vi "Get SMO Database Paths.vi"(5 "getAll Cluster":variant, 7 "Default Paths":string, 8 "error in (no error)":errorcluster, 11 "instrument.PPMS in":refnum<class "instrument.PPMS1.lvclass">) -> (0 "error out":errorcluster, 2 "Paths":string, 3 "instrument.PPMS out":refnum<class "instrument.PPMS1.lvclass">)   [LabVIEW 2019, in "instrument.PPMS1.lvclass"]
uses:
  instrument.PPMS1.lvclass
  instrument.PPMS/instrument.PPMS.lvclass
  instrument.PPMS/Typedefs/PPMS.getAll--cluster.ctl
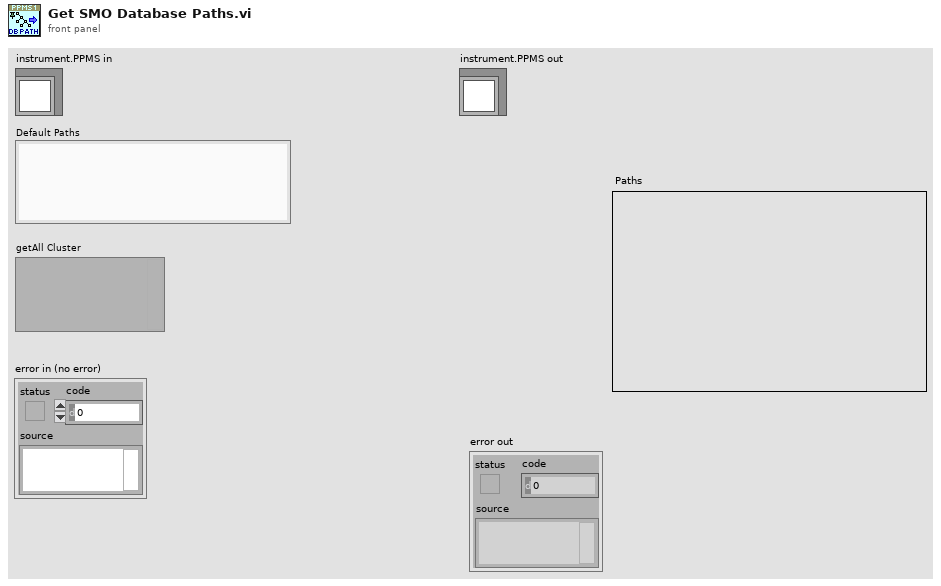
[diagram p1: front panel]
types:
  T1 = typedef "instrument.PPMS.lvclass/PPMS.getAll--cluster.ctl" = cluster{"Chamber Status":string, "Helium Level":dbl, "Temperature":dbl, "Temperature Status":string, "Magnetic Field":dbl, "Magnet Status":string, "Position":dbl}
  T2 = cluster{"Chamber Status":string, "Helium Level":dbl, "Temperature":dbl, "Temperature Status":string, "Magnetic Field":dbl, "Magnet Status":string}
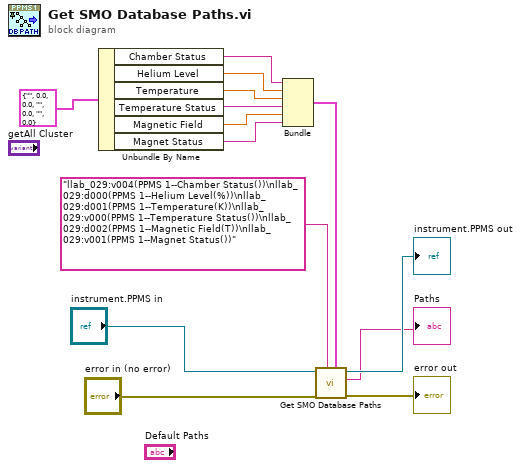
[diagram p0: block diagram]
diagram:
  n1 = Unbundle By Name(T1 {"Chamber Status"="", "Helium Level"=0.0, "Temperature"=0.0, "Temperature Status"="", "Magnetic Field"=0.0, "Magnet Status"="", "Position"=0.0} ("getAll")) -> ("Chamber Status"=w2:string, "Helium Level"=w5:dbl, "Temperature"=w6:dbl, "Temperature Status"=w7:string, "Magnetic Field"=w4:dbl, "Magnet Status"=w3:string)
  n2 = Bundle("Chamber Status"=w2, "Helium Level"=w5, "Temperature"=w6, "Temperature Status"=w7, "Magnetic Field"=w4, "Magnet Status"=w3) -> (w1:T2)  [unwired: 1 in]
  n3 = call-parent "Get SMO Database Paths.vi"("getAll Cluster"=w1, "Default Paths"="llab_029:v004(PPMS 1--Chamber Status())\nllab_029:d000(PPMS 1--Helium Level(%))\nllab_029:d001(PPMS 1--Temperature(K))\nllab_029:v000(PPMS 1--Temperature Status())\nllab_029:d002(PPMS 1--Magnetic Field(T))\nllab_029:v001(PPMS 1--Magnet Status())" ("Paths"), "error in (no error)"="error in (no error)", "instrument.PPMS in"="instrument.PPMS in") -> ("error out"=→"error out":errorcluster, "Paths"=→"Paths":string, "instrument.PPMS out"=→"instrument.PPMS out":refnum<class "instrument.PPMS1.lvclass">)  [unwired: 5 in]
